vi "CXNN.vi"(11 "Variables and Memory in":T1 {"GFX" format="%02x"}) -> (3 "Variables and Memory out":T1 {"GFX" format="%02x"})   [LabVIEW 2021]
uses:
  Controls/ClusterF.ctl
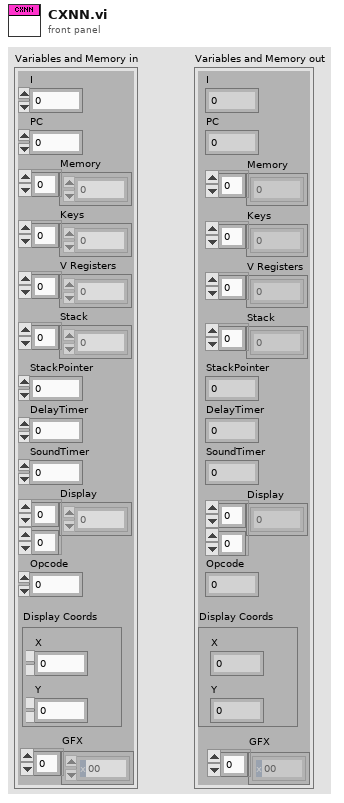
[diagram p1: front panel]
types:
  T1 = typedef "ClusterF.ctl" = cluster{"I":u16, "PC":u16, "Memory":u8[], "Keys":u8[], "V Registers":u8[], "Stack":u16[], "StackPointer":u16, "DelayTimer":u8, "SoundTimer":u8, "Display":u8[][], "Opcode":u16, "Display Coords":cluster{"X":u8, "Y":u8}, "GFX":u8[]}
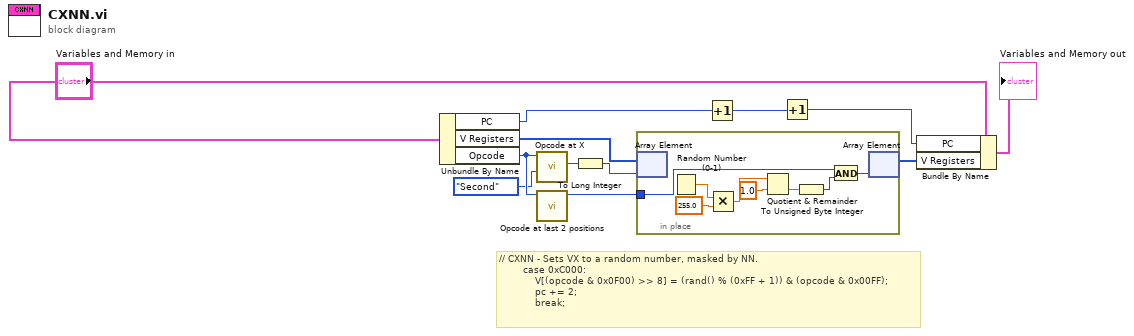
[diagram p0: block diagram]
diagram:
  # "// CXNN - Sets VX to a random number, masked by NN.\n        case 0xC000:\n            V[(opcode & 0x0F00) >> 8] = (rand() % (0xFF + 1)) & (opcode & 0x00FF);\n            pc += 2;\n            break;"
  n1 = Unbundle By Name("Variables and Memory in") -> ("PC"=w3:u16, "V Registers"=w8:u8[], "Opcode"=w7:u16)
  n2 = call "Opcode at X.vi"("X Position"=enum16{"First", "Second", "Third", "Fourth"}."Second", "Opcode"=w7) -> ("Opcode at X Position (U8)"=w9:u8)  [unwired: 9 in]
  n3 = call "Opcode at last 2 positions.vi"("Opcode"=w7) -> ("00FF"=w11:u8)  [unwired: 10 in]
  n4 = To Long Integer(number=w9) -> (32bit integer=w10:i32)
  n5 = in-place {
    in-place-border: w11 -> [w18]
    n6 = in-place-array #1(w8, w10) -> ()  [unwired: 1 out]
    n7 = Random Number (0-1)() -> (number: 0 to 1=w20:dbl)
    n8 = Multiply(x=w20, y=255.0) -> (x*y=w15:dbl)
    n9 = Quotient & Remainder(x=w15, y=1.0) -> (floor(x/y)=w13:dbl)  [unwired: 1 out]
    n10 = To Unsigned Byte Integer(number=w13) -> (unsigned 8bit integer=w17:u8)
    n11 = And(x=w18, y=w17) -> (x .and. y?=w16:u8)
    n12 = in-place-array #1(w16) -> (w12:u8[])  [unwired: 1 out]
  }
  n13 = Increment(x=w3) -> (x+1=w4:u16)
  n14 = Increment(x=w4) -> (x+1=w5:u16)
  n15 = Bundle By Name(cluster="Variables and Memory in", "PC"=w5, "V Registers"=w12) -> (→"Variables and Memory out":T1)
